vi "libssh2_sftp_get_channel.vi"(8 "error in (no error)":errorcluster, 11 "sftp":T2) -> (0 "error out":errorcluster, 3 "channel":T1)   [LabVIEW 2013, in "libssh2.lvlib"]
doc: "Get the channel associated with an SFTP session."
uses:
  libssh2.lvlib
  SFTP Refnum.ctl
  Channel Refnum.ctl
  Not An SFTP Refnum.vi
  <vilib>/Utility/error.llb/Error Cluster From Error Code.vi
  Global Settings.vi
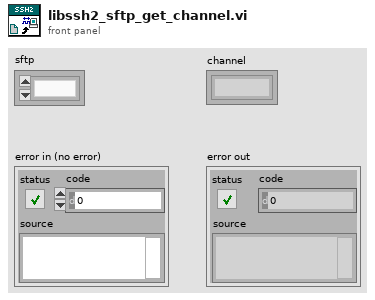
[diagram p1: front panel]
types:
  T1 = typedef "libssh2.lvlib/Channel Refnum.ctl" = refnum<k1>
  T2 = typedef "libssh2.lvlib/SFTP Refnum.ctl" = refnum<k1>
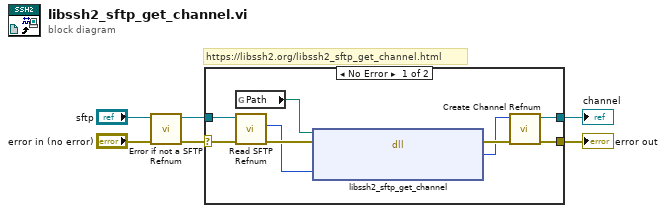
[diagram p0: block diagram]
diagram:
  # "https://libssh2.org/libssh2_sftp_get_channel.html"
  n1 = call "Error if not a SFTP Refnum.vi"("error in (no error)"="error in (no error)", "sftp"="sftp") -> ("error out"=w5:errorcluster, "sftp out"=w4:T2)  [unwired: 8 in]
  n2 = case shown="No Error" w5 {
    selector: w5 -> [w14 w16]
    tunnel: w4 -> [w13 _]
    tunnel: [w9 w16] -> w3
    tunnel: [w7 _] -> w1
    frame No Error {
      n3 = global read "Global Settings.vi" "Path"() -> (w15:path)
      n4 = call "Read SFTP Refnum.vi"("error in (no error)"=w14, "sftp"=w13) -> ("error out"=w12:errorcluster, "LIBSSH2_SFTP*"=w11:u64)  [unwired: 8 in]
      n5 = dll-call lib="?" fn="libssh2_sftp_get_channel"(path in=w15, error in=w12, "sftp"=w11) -> (error out=w10:errorcluster, "return value"=w8:u64)  [unwired: 2 in, 1 out]
      n6 = call "Create Channel Refnum.vi"("error in (no error)"=w10, "LIBSSH2_CHANNEL*"=w8) -> ("error out"=w9:errorcluster, "channel"=w7:T1)  [unwired: 8 in]
    }
    frame Error {
    }
  }
  "error out" <- w3
  "channel" <- w1
